vi "EnterSampleNameDialog.vi"(8 "Error In":errorcluster) -> (0 "Error Out":errorcluster, 2 "Schedule File out":path, 3 "Sample Name":string)   [LabVIEW 2019]
panel:
  in  "Schedule File":path
  in  "Next":bool
  in  "Sample Name":string
  # "Enter Sample Plan"
  # "Enter the name of the sample using no spaces or underscores - they will be automatically removed! Select the schedule file to be used"
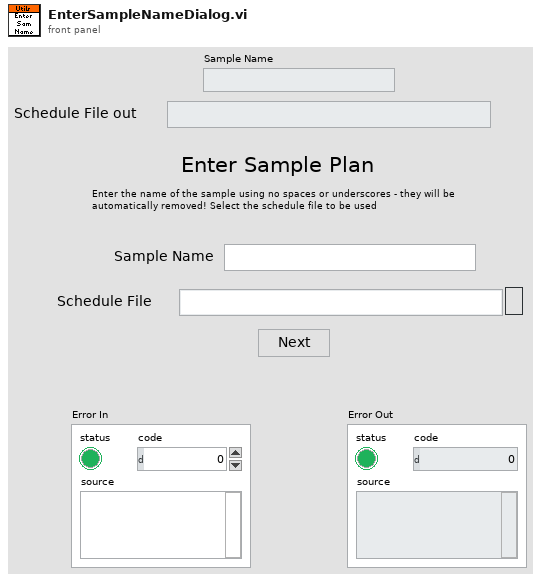
[diagram p1: front panel]
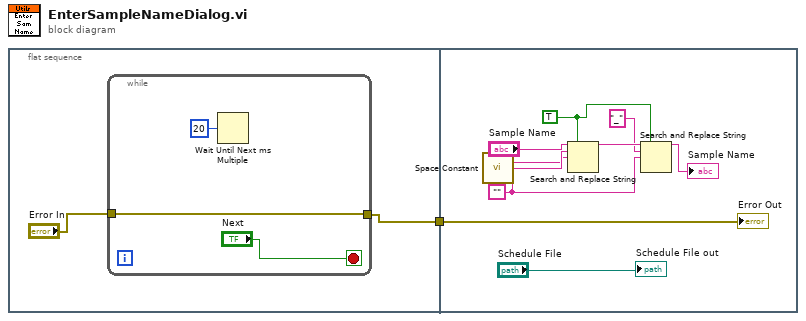
[diagram p0: block diagram]
diagram:
  n1 = flat-sequence {
    tunnel: [w2] -> w1
    tunnel: w1 -> [w15]
    frame #0 {
      n2 = while {
        tunnel: [w4] -> w2
        tunnel: "Error In" -> [w4]
        stop <- "Next" stop-if-true
        n3 = Wait Until Next ms Multiple(millisecond multiple=u32 20) -> ()  [unwired: 1 out]
      }
    }
    frame #1 {
      w9 = TRUE ("replace all? (F)")
      w10 = ""
      n4 = call <vilib>:"Space Constant.vi"() -> ("String"=w13:string)
      n5 = Search and Replace String(replace all?=w9, input string="Sample Name", search string=w13, replace string=w10) -> (result string=w12:string)  [unwired: 4 in, 3 out]
      n6 = Search and Replace String(replace all?=w9, input string=w12, search string="_" ("substring (\"\")"), replace string=w10) -> (result string=→"Sample Name":string)  [unwired: 4 in, 3 out]
      "Error Out" <- w15
      "Schedule File out" <- "Schedule File"
    }
  }
